vi "Kinematics (SubVI).vi"(0 "Forward Left":dbl, 1 "Forward Right":dbl, 2 "Back Left":dbl, 3 "Back Right":dbl) -> (7 "X":dbl, 8 "Y":dbl)   [LabVIEW 2017]
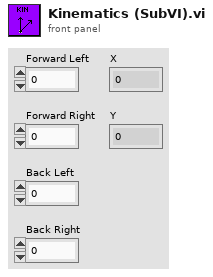
[diagram p1: front panel]
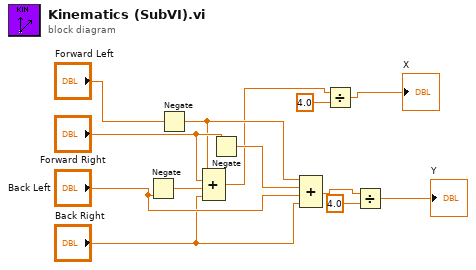
[diagram p0: block diagram]
diagram:
  n1 = Negate(x="Back Left") -> (-x=w7:dbl)
  n2 = Negate(x="Forward Left") -> (-x=w8:dbl)
  n3 = Compound Arithmetic op=ADD(w8, "Forward Right", w7, "Back Right") -> (w5:dbl)
  n4 = Negate(x="Forward Right") -> (-x=w9:dbl)
  n5 = Compound Arithmetic op=ADD(w8, w9, "Back Left", "Back Right") -> (w2:dbl)
  n6 = Divide(x=w5, y=4.0) -> (x/y=→"X":dbl)
  n7 = Divide(x=w2, y=4.0) -> (x/y=→"Y":dbl)
